vi "ComputeChecksum.vi"(10 "Input Command":string) -> (1 "Checksum":string, 2 "Command Message":string)   [LabVIEW 2017, in "Thermal Shock.lvlib"]
uses:
  Thermal Shock.lvlib
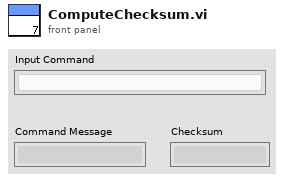
[diagram p1: front panel]
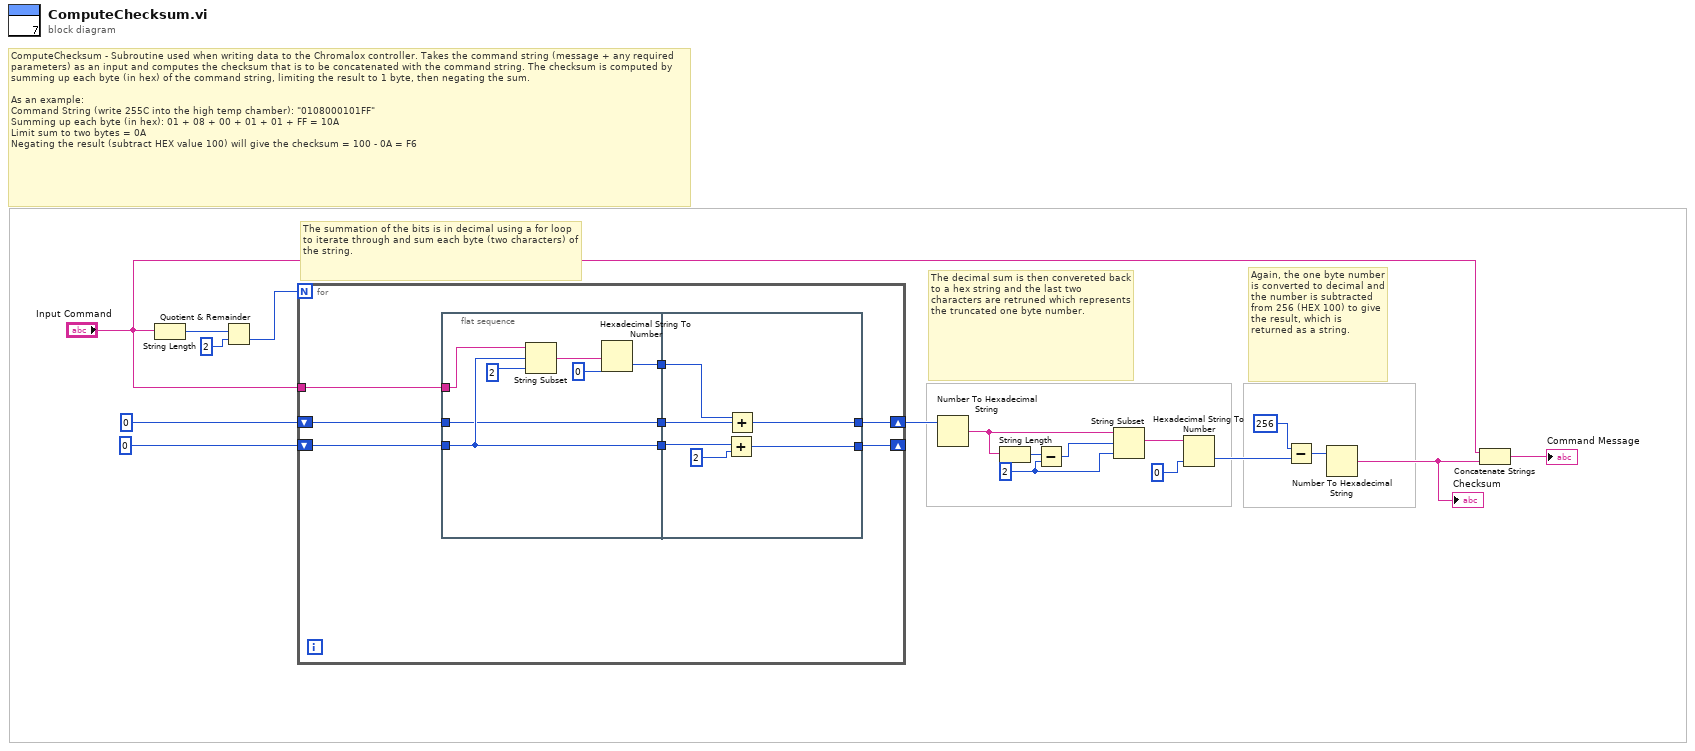
[diagram p0: block diagram]
diagram:
  w4 = 2
  # "Again, the one byte number is converted to decimal and the number is subtracted from 256 (HEX 100) to give the result, which is returned as a string."
  # "The decimal sum is then convereted back to a hex string and the last two characters are retruned which represents the truncated one byte number."
  # "The summation of the bits is in decimal using a for loop to iterate through and sum each byte (two characters) of the string."
  # "ComputeChecksum - Subroutine used when writing data to the Chromalox controller. Takes the command string (message + any required parameters) as an input and computes the checksum that is to be concatenated with the command string. The checksum is computed by summing up each byte (in hex) of the command string, limiting the result to 1 byte, then negating the sum.  \n\nAs an example: \nCommand String (write 255C into the high temp chamber): \"0108000101FF\"\nSumming up each byte (in hex): 01 + 08 + 00 + 01 + 01 + FF = 10A\nLimit sum to two bytes = 0A\nNegating the result (subtract HEX value 100) will give the checksum = 100 - 0A = F6"
  n1 = String Length(string="Input Command") -> (length=w18:i32)
  n2 = Quotient & Remainder(x=w18, y=2) -> (floor(x/y)=w16:i32)  [unwired: 1 out]
  n3 = for {
    N: w16 -> [_]
    tunnel: "Input Command" -> [w23]
    shift-right: [w24] -> _
    shift-left: 0 -> [w26]
    shift-right: [w19] -> w13
    shift-left: u16 0 -> [w21]
    n4 = flat-sequence {
      tunnel: w26 -> [w32]
      tunnel: [w32] -> w25
      tunnel: w23 -> [w31]
      tunnel: [w28] -> w22
      tunnel: w21 -> [w27]
      tunnel: [w27] -> w20
      tunnel: w25 -> [w39]
      tunnel: [w37] -> w24
      tunnel: w22 -> [w34]
      tunnel: w20 -> [w35]
      tunnel: [w36] -> w19
      frame #0 {
        n5 = String Subset(string=w31, offset (0)=w32, length (rest)=2) -> (substring=w30:string)
        n6 = Hexadecimal String To Number(string=w30, default (0uL)=u16 0) -> (number=w28:u16)  [unwired: 1 in, 1 out]
      }
      frame #1 {
        n7 = Add(x=w39, y=2) -> (x+y=w37:i32)
        n8 = Add(x=w34, y=w35) -> (x+y=w36:u16)
      }
    }
  }
  n9 = Number To Hexadecimal String(2:w13) -> (0:w7:string)  [unwired: 1 in]
  n10 = String Length(string=w7) -> (length=w6:i32)
  n11 = Subtract(x=w6, y=w4) -> (x-y=w5:i32)
  n12 = String Subset(string=w7, offset (0)=w5, length (rest)=w4) -> (substring=w12:string)
  n13 = Hexadecimal String To Number(string=w12, default (0uL)=u16 0) -> (number=w9:u16)  [unwired: 1 in, 1 out]
  n14 = Subtract(x=u16 256, y=w9) -> (x-y=w8:u16)
  n15 = Number To Hexadecimal String(2:w8) -> (0:w1:string)  [unwired: 1 in]
  "Checksum" <- w1
  n16 = Concatenate Strings("Input Command", w1) -> (→"Command Message":string)
